vi "Update Channel Monitor Listbox.vi"(8 "error in (no error)":errorcluster, 10 "Input Channels":T1[](array[typedef]) {"Node Ref" format="%.0x"}, 11 "Monitored Channels":refnum<vi>) -> (0 "error out":errorcluster)   [LabVIEW 2019, in "Protection and Counter Support System Explorer.lvlib"]
uses:
  Protection and Counter Support System Explorer.lvlib
  Types/Protection Signal Linked Channel.ctl
  <vilib>/NI VeriStand/Custom Device API/Custom Device Item Ref.ctl
  <vilib>/NI VeriStand/Custom Device API/Custom Device API.lvlib
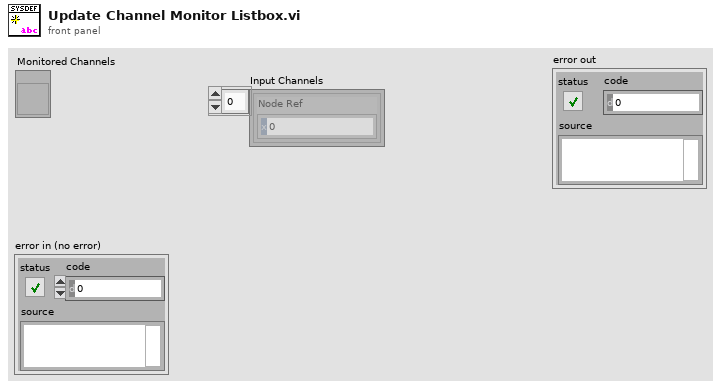
[diagram p1: front panel]
types:
  T1 = typedef "Protection and Counter Support System Explorer.lvlib/Protection Signal Linked Channel.ctl" = cluster{"Node Ref":T2}
  T2 = typedef "Custom Device API.lvlib/Custom Device Item Ref.ctl" = u64
  T3 = typedef "Custom Device API.lvlib/Custom Device Item Info.ctl" = cluster{"Name":string, "Is Channel":bool, "GUID":string, "Is Waveform":bool}
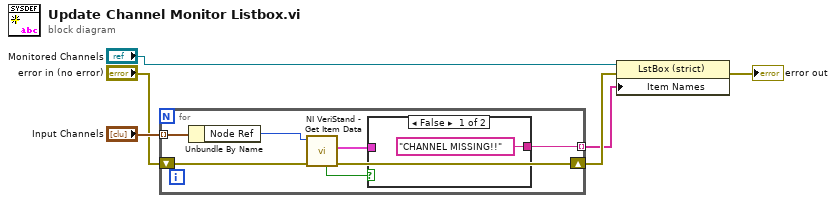
[diagram p0: block diagram]
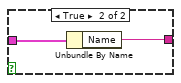
[diagram p2: hidden frame]
diagram:
  n1 = for {
    tunnel: "Input Channels" -> [w13] mode=indexing
    shift-right: [w10] -> w2
    shift-left: "error in (no error)" -> [w11]
    tunnel: [w8] -> w1 mode=indexing
    n2 = Unbundle By Name(w13) -> ("Node Ref"=w12:T2)
    n3 = call <vilib>:"NI VeriStand - Get Item Data.vi"("error in (no error)"=w11, "Item Ref in"=w12) -> ("error out"=w10:errorcluster, "Item Info"=w9:T3, "Found"=w7:bool)  [unwired: 6 in, 1 out]
    n4 = case shown="False" w7 {
      tunnel: w9 -> [_ w16]
      tunnel: ["CHANNEL MISSING!!" ("Name") w15] -> w8
      frame False {
      }
      frame True {
        n5 = Unbundle By Name(w16) -> ("Name"=w15:string)
      }
    }
  }
  n6 = property class="LstBox (strict)"(reference="Monitored Channels", error in=w2, "Item Names"=w1) -> (error out=→"error out":errorcluster)  [unwired: 1 out]
